vi "OEE_SCREEN_1_calculate_quality_yeild.vi"(2 "rejects":string, 3 "actual":string) -> (0 "quality_yeild":string)   [LabVIEW 2019]
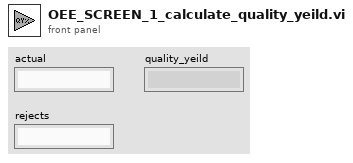
[diagram p1: front panel]
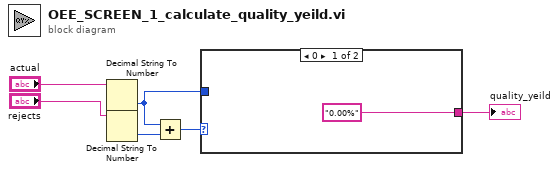
[diagram p0: block diagram]
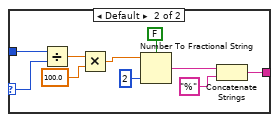
[diagram p2: hidden frame]
diagram:
  n1 = Decimal String To Number(string="actual") -> (number=w6:i32)  [unwired: 2 in, 1 out]
  n2 = Decimal String To Number(string="rejects") -> (number=w3:i32)  [unwired: 2 in, 1 out]
  n3 = Add(x=w6, y=w3) -> (x+y=w4:i32)
  n4 = case shown="0" w4 {
    selector: w4 -> [_ w16]
    tunnel: ["0.00%" w8] -> w5
    tunnel: w6 -> [_ w17]
    frame 0 {
    }
    frame Default {
      n5 = Divide(x=w17, y=w16) -> (x/y=w14:dbl)
      n6 = Multiply(x=w14, y=100.0) -> (x*y=w12:dbl)
      n7 = Number To Fractional String(use system decimal point (T)=FALSE, number=w12, precision (6)=i16 2) -> (F-format string=w10:string)  [unwired: 1 in]
      n8 = Concatenate Strings(w10, "%" ("string")) -> (w8:string)
    }
  }
  "quality_yeild" <- w5
